vi "Fit Model to Plot v3.vi"(0 "Fit Plot Information":T9={"XY Graph Ref"=refnum, "Mouse Coordinates"={"X"=0.0, "Y"=0.0}, "Fit Model"=enum."Select a Fit Model...", "Plot Index"=-1}, 5 "Fit Settings":T2={"Use Original Plot # Points"=TRUE, "# Fit Plot Points"=0, "Fitting Method"=enum."Least Square", "Weighted Fit"=enum."1/Variance (Neyman)", "Show All Fit Components"=FALSE, "Axis Type"=0, "Show Fit Residuals"=TRUE, "Residual Type"=enum."Standard", "Fitting Algorithm"=enum."Levenberg-Marquardt", "Show Confidence Interval"=TRUE, "Confidence Level"=95.0} {"Confidence Level" min=0.0 max=100.0; "Axis Type" items=["Linear", "Logarithmic"]}, 7 "Additional Parameters (in)":variant, 9 "Fixed Parameters":T8, 11 "error in (no error)":errorcluster, 12 "Termination Criteria":T1={"Max Iterations"=1000, "Max Function Calls"=10000, "Max Time"=1000.0, "Function Tolerance"=1e-09, "Parameter Tolerance"=1e-09, "Gradient Tolerance"=1e-09, "Min Lambda"=1e-09, "Max Lambda"=1000000000.0, "Initial Tick Count"=0}, 13 "Send Graph to Notebook? (F)":bool) -> (1 "Fitted Plot":cluster{"X Array":dbl[], "Y Array":dbl[]}, 2 "Graph Name":string, 3 "Plot Name":string, 4 "Best Fit":dbl[](array[numeric]), 6 "Fit Parameter Names":string[](array[string]), 8 "Additional Parameters (out)":variant, 10 "Fit Parameter Values":dbl[](array[numeric]), 14 "Fit Result String":string, 15 "error out":errorcluster)   [LabVIEW 2021, in "Fits.lvlib"]
uses:
  Fits.lvlib
  Fit Plot Request Information.ctl
  <vilib>/Utility/miscctls.llb/LVPointDoubleTypeDef.ctl
  Fit Models.ctl
  D-Only Fixed Parameters.ctl
  Fit Settings.ctl
  Nonlinear Fit Method.ctl
  Ramp Type.ctl
  Residual Type.ctl
  Non-linear Fitting Algorithm.ctl
  My Fit Stopping Criteria.ctl
  Error/Error.lvlib
  Graphs/XY Graph/XY Graph Add-Ons.lvlib
  IRF(X)PSED/Fit Weights Type v2.ctl
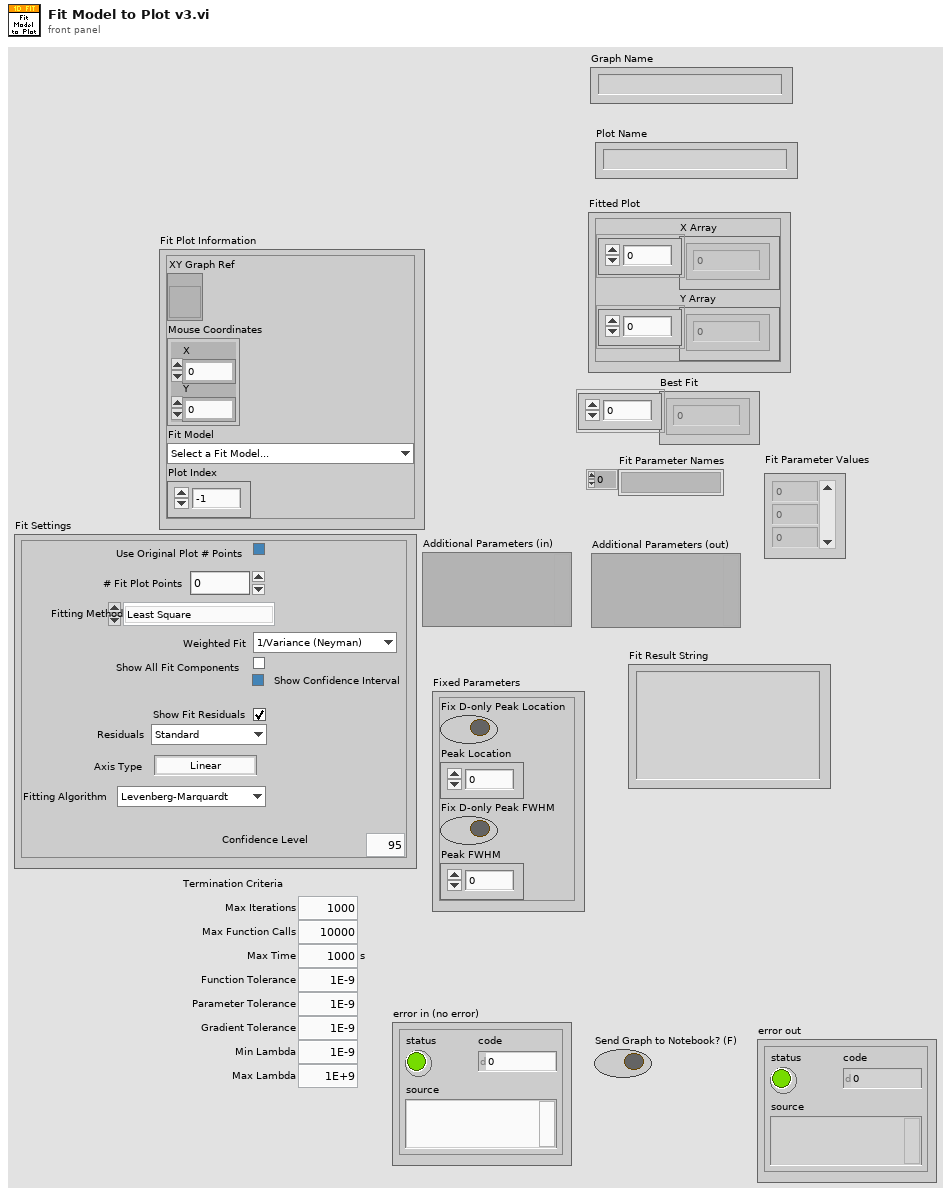
[diagram p1: front panel]
types:
  T1 = typedef "Fits.lvlib/My Fit Stopping Criteria.ctl" = cluster{"Max Iterations":i32, "Max Function Calls":i32, "Max Time":dbl[unit], "Function Tolerance":dbl, "Parameter Tolerance":dbl, "Gradient Tolerance":dbl, "Min Lambda":dbl, "Max Lambda":dbl, "Initial Tick Count":u32}
  T2 = typedef "Fits.lvlib/Fit Settings.ctl" = cluster{"Use Original Plot # Points":bool, "# Fit Plot Points":u32, "Fitting Method":T3, "Weighted Fit":T4, "Show All Fit Components":bool, "Axis Type":T5, "Show Fit Residuals":bool, "Residual Type":T6, "Fitting Algorithm":T7, "Show Confidence Interval":bool, "Confidence Level":dbl}
  T3 = typedef "Fits.lvlib/Nonlinear Fit Method.ctl" = enum16{"Least Square", "Least Absolute Residual", "Bisquare", "MLE"}
  T4 = typedef "Fits.lvlib/Fit Weights Type v2.ctl" = enum16{"Unweighted", "1/Variance (Neyman)", "1/Variance (Pearson)", "Best of All"}
  T5 = typedef "Fits.lvlib/Ramp Type.ctl" = u16
  T6 = typedef "Fits.lvlib/Residual Type.ctl" = enum16{"Standard", "Normalized", "Reduced"}
  T7 = typedef "Fits.lvlib/Non-linear Fitting Algorithm.ctl" = enum16{"Levenberg-Marquardt", "Trust-Region Dogleg"}
  T8 = typedef "Fits.lvlib/D-Only Fixed Parameters.ctl" = cluster{"Fix D-only Peak Location":bool, "Peak Location":dbl, "Fix D-only Peak FWHM":bool, "Peak FWHM":dbl}
  T9 = typedef "Fits.lvlib/Fit Plot Request Information.ctl" = cluster{"XY Graph Ref":refnum<vi>, "Mouse Coordinates":T10, "Fit Model":T11, "Plot Index":i32}
  T10 = typedef "LVPointDoubleTypeDef.ctl" = cluster{"X":dbl, "Y":dbl}
  T11 = typedef "Fits.lvlib/Fit Models.ctl" = enum16{"Select a Fit Model...", "           Single Peak", "Gaussian", "Asymmetric Gaussian", "Lorentzian", "Asymmetric Lorentzian", "Gaussian/Lorentzian", "Lorentzian/Gaussian", "           Double Peak", "Two Gaussians", "Two Asymmetric Gaussians", "Two H-Connected Gaussians", "Two T-Connected Gaussians", "Two H-Connected Asymmetric Gaussians", "Two T-Connected Asymmetric Gaussians", "           Triple Peak", "Three Gaussians", "Three Asymmetric Gaussians", "              Decays", "1-Exponential", "IRF*PSED", "2-Exponentials", "            Power Law", "Power Law", "Power Law with Offset", "               ACF", "2D Gaussian ACF", "2D Gaussian + Blinking ACF", "2D Gaussian + Flow ACF", "3D Gaussian ACF", "3D Gaussian + Blinking ACF", "             Multiplot", "2D Gaussian ACF & 2D Gaussian + Flow ACF"}
  T12 = typedef "XY Graph Add-Ons.lvlib/XY Graph Refnum.ctl" = refnum<vi>
  T13 = typedef "Fits.lvlib/Fit Model Information.ctl" = cluster{"Fit Model":T11, "LM Function & Gradient":refnum<vi>, "Additional Fit Settings":variant}
  T14 = typedef "Fits.lvlib/Fit Output Data.ctl" = cluster{"Fit Parameters Cluster":variant, "Fit Parameters Uncertainties Cluster":variant, "Additional Data":variant}
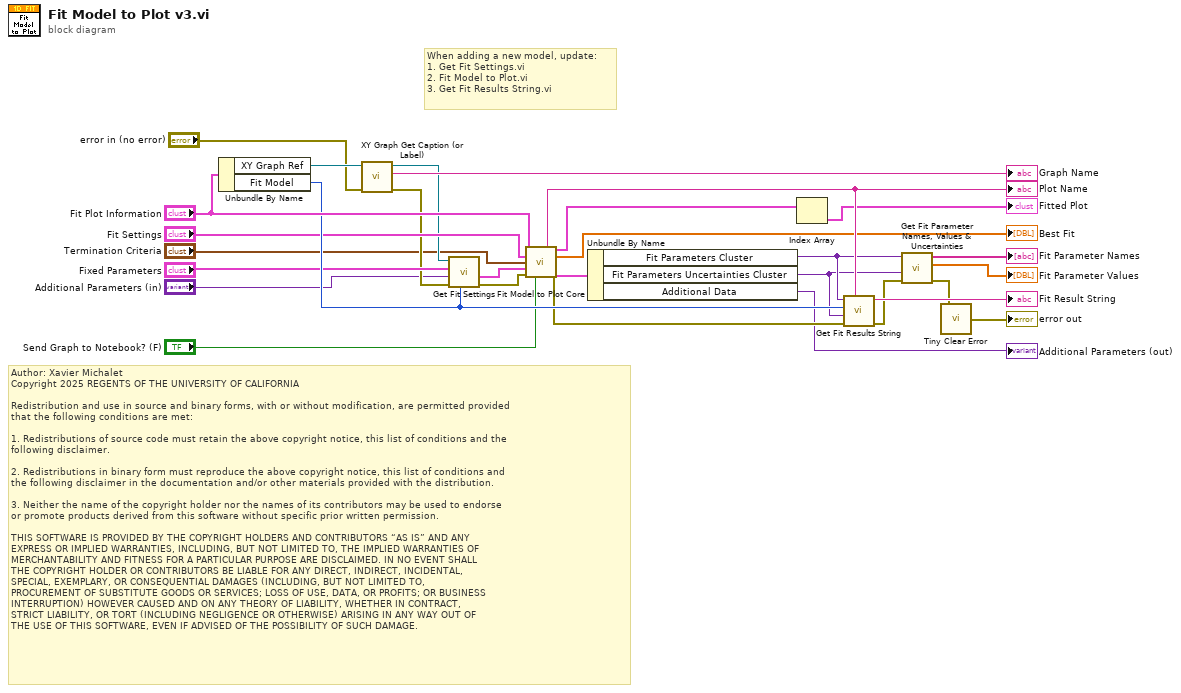
[diagram p0: block diagram]
diagram:
  # "Author: Xavier Michalet\nCopyright 2025 REGENTS OF THE UNIVERSITY OF CALIFORNIA\n\nRedistribution and use in source and binary forms, with or without modification, are permitted provided\nthat the following conditions are met:\n\n1. Redistributions of source code must retain the above copyright notice, this list of conditions and the\nfollowing disclaimer.\n\n2. Redistributions in binary form must reproduce the above copyright notice, this list of conditions and\nthe following disclaimer in the documentation and/or other materials provided with the distribution.\n\n3. Neither the name of the copyright holder nor the names of its contributors may be used to endorse \nor promote products derived from this software without specific prior written permission.\n\nTHIS SOFTWARE IS PROVIDED BY THE COPYRIGHT HOLDERS AND CONTRIBUTORS “AS IS” AND ANY \nEXPRESS OR IMPLIED WARRANTIES, INCLUDING, BUT NOT LIMITED TO, THE IMPLIED WARRANTIES OF\nMERCHANTABILITY AND FITNESS FOR A PARTICULAR PURPOSE ARE DISCLAIMED. IN NO EVENT SHALL\nTHE COPYRIGHT HOLDER OR CONTRIBUTORS BE LIABLE FOR ANY DIRECT, INDIRECT, INCIDENTAL, \nSPECIAL, EXEMPLARY, OR CONSEQUENTIAL DAMAGES (INCLUDING, BUT NOT LIMITED TO, \nPROCUREMENT OF SUBSTITUTE GOODS OR SERVICES; LOSS OF USE, DATA, OR PROFITS; OR BUSINESS\nINTERRUPTION) HOWEVER CAUSED AND ON ANY THEORY OF LIABILITY, WHETHER IN CONTRACT, \nSTRICT LIABILITY, OR TORT (INCLUDING NEGLIGENCE OR OTHERWISE) ARISING IN ANY WAY OUT OF\nTHE USE OF THIS SOFTWARE, EVEN IF ADVISED OF THE POSSIBILITY OF SUCH DAMAGE."
  # "When adding a new model, update:\n1. Get Fit Settings.vi\n2. Fit Model to Plot.vi\n3. Get Fit Results String.vi"
  n1 = Unbundle By Name("Fit Plot Information") -> ("XY Graph Ref"=w17:refnum<vi>, "Fit Model"=w22:T11)
  n2 = call "XY Graph Get Caption (or Label).vi"("error in (no error)"="error in (no error)", "XY Graph in"=w17) -> ("error out"=w13:errorcluster, "Caption (or Label) Text"=→"Graph Name":string, "XY Graph out"=w14:T12)  [unwired: 7 in]
  n3 = call "Get Fit Settings.vi"("Fit Model"=w22, "Error In"=w13, "Additional Parameters"="Additional Parameters (in)", "Fixed Parameters"="Fixed Parameters", "XY Graph Ref"=w14) -> ("Error Out"=w19:errorcluster, "Fit Model Information"=w7:T13)  [unwired: 3 in, 2 out]
  n4 = call "Fit Model to Plot Core.vi"("Fit Plot Information"="Fit Plot Information", "Fit Settings"="Fit Settings", "Termination Criteria"="Termination Criteria", "Fit Model Information"=w7, "error in (no error)"=w19, "Send Graph to Notebook?"="Send Graph to Notebook? (F)") -> ("Plot Name"=w24:string, "Array of Plots (Fit, Components, Residuals)"=w25:cluster{"X Array":dbl[], "Y Array":dbl[]}[], "best nonlinear fit"=→"Best Fit":dbl[], "Fit Output Data"=w6:T14, "error out"=w4:errorcluster)  [unwired: 4 in, 1 out]
  "Plot Name" <- w24
  n5 = Unbundle By Name(w6) -> ("Fit Parameters Cluster"=w5:variant, "Fit Parameters Uncertainties Cluster"=w2:variant, "Additional Data"=→"Additional Parameters (out)":variant)
  n6 = Index Array(array=w25) -> (element=→"Fitted Plot":cluster{"X Array":dbl[], "Y Array":dbl[]})  [unwired: 1 in]
  n7 = call "Get Fit Results String.vi"("Plot Name"=w24, "error in (no error)"=w4, "Fit Parameters Uncertainties Cluster"=w2, "Fit Model"=w22, "Fit Parameters Cluster"=w5) -> ("error out"=w3:errorcluster, "Fit Results String"=→"Fit Result String":string)  [unwired: 5 in]
  n8 = call "Get Fit Parameter Names, Values & Uncertainties.vi"("error in (no error)"=w3, "Fit Parameter Uncertainties"=w2, "Fit Parameters"=w5) -> ("Error Out"=w23:errorcluster, "Fit Parameter Values"=→"Fit Parameter Values":dbl[], "Fit Parameter Names"=→"Fit Parameter Names":string[])  [unwired: 5 in, 1 out]
  n9 = call "Tiny Clear Error.vi"("Error In"=w23) -> ("no Error Out"=→"error out":errorcluster)  [unwired: 8 in]
